vi "waitOnListener.vi"(8 "error in (no error)":errorcluster, 11 "TCPServer in":refnum<class "TCPServer.lvclass">) -> (0 "error out":errorcluster, 2 "remote address":string, 3 "TCPServer out":refnum<class "TCPServer.lvclass">)   [LabVIEW 2016, in "TCPServer.lvclass"]
uses:
  TCPServer.lvclass
  C:/Users/aanania/Documents/ss_atdome/ts_labview_tcp/TCPCommunicator/TCPCommunicator.lvclass
  TCPCommunicator/TCPCommunicator.lvclass/TCPCommunicator.ctl
  TCPSettings/TCPSettings.lvclass
  TCPCommunicator/TCPCommunicator.lvclass
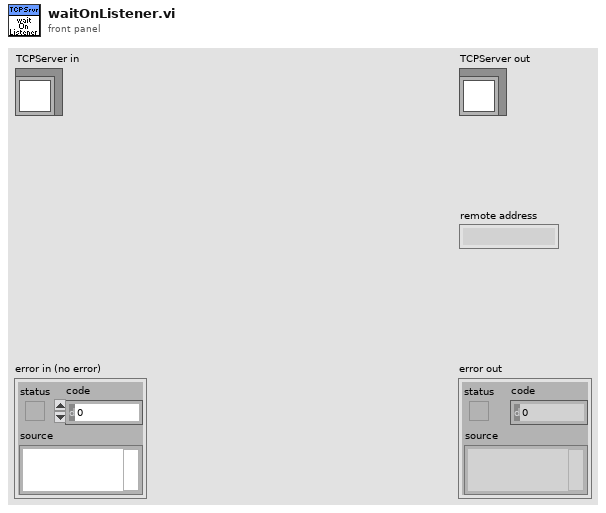
[diagram p1: front panel]
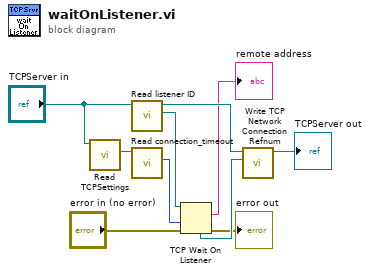
[diagram p0: block diagram]
diagram:
  n1 = call-dynamic "Read TCPSettings.vi"("TCPCommunicator in"="TCPServer in") -> ("TCPSettings.lvclass"=w5:refnum<class "TCPSettings.lvclass">)  [unwired: 8 in, 2 out]
  n2 = call "Read listener ID.vi"("TCPCommunicator in"="TCPServer in") -> ("listener ID"=w10:refnum<k5>, "TCPCommunicator out"=w9:refnum<class "TCPServer.lvclass">)  [unwired: 8 in, 1 out]
  n3 = call-dynamic "Read connection_timeout .vi"("TCPSettings in"=w5) -> ("connection_timeout"=w6:i32)  [unwired: 8 in, 2 out]
  n4 = TCP Wait On Listener(8:"error in (no error)", 9:w6, 11:w10) -> (0:→"error out":errorcluster, 2:→"remote address":string, 4:w8:refnum<k5>)  [unwired: 3 out]
  n5 = call-dynamic "Write TCP Network Connection Refnum.vi"("TCP Network Connection Refnum"=w8, "TCPCommunicator in"=w9) -> ("TCPCommunicator out"=→"TCPServer out":refnum<class "TCPServer.lvclass">)  [unwired: 8 in, 1 out]
